vi "配置文件保存.vi"   [LabVIEW 2022 SP3, in "斯坦道CODMn.lvlib"]
uses:
  <vilib>/Utility/config.llb/NI_LVConfig.lvlib
  <userlib>/_OpenG.lib/variantconfig/variantconfig.llb/openg_variant_configuration_file.lvlib
types:
  T1 = typedef "NI_LVConfig.lvlib/Config Data RefNum.ctl" = refnum<k1>
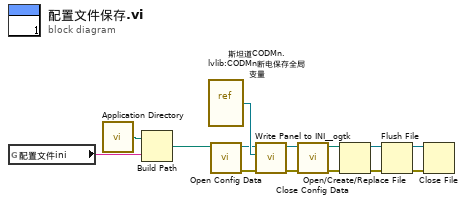
[diagram p0: block diagram]
diagram:
  n1 = global read "COD内部交互全局.vi" "配置文件ini"() -> (w2:string)
  n2 = call <vilib>:"Application Directory.vi"() -> ("Application Directory"=w1:path)
  n3 = Build Path(base path=w1, name or relative path=w2) -> (appended path=w14:path)
  n4 = vi-ref "斯坦道CODMn.lvlib:CODMn断电保存全局变量.vi"() -> (w4:refnum<vi>)
  n5 = call <vilib>:"Open Config Data.vi"("configuration file path"=w14) -> ("error out"=w6:errorcluster, "refnum"=w3:T1)  [unwired: 8 in, 1 out]
  n6 = call <userlib>:"Write Panel to INI__ogtk.vi"("error in (no error)"=w6, "VI ref"=w4, "refnum"=w3) -> ("error out"=w7:errorcluster, "refnum out"=w5:T1)  [unwired: 7 in]
  n7 = call <vilib>:"Close Config Data.vi"("error in (no error)"=w7, "refnum"=w5) -> ("error out"=w12:errorcluster, "file path"=w13:path)  [unwired: 8 in]
  n8 = Open/Create/Replace File(file path (use dialog)=w13, error in=w12) -> (refnum out=w9:refnum<file>, error out=w8:errorcluster)  [unwired: 4 in, 1 out]
  n9 = Flush File(refnum=w9, error in=w8) -> (refnum out=w10:refnum<file>, error out=w11:errorcluster)
  n10 = Close File(refnum=w10, error in=w11) -> ()  [unwired: 2 out]
